vi "Begin.vi"(8 "error in":errorcluster) -> (0 "error out":errorcluster)   [LabVIEW 2014]
doc: "Called before other user functions, this VI is expected to open initial I/O refnums, load in file data, and do all program initialization. Notice that the <B>error out</B> terminal is simply used for data flow. Wiring it to other structures or subVIs ensures that this VI runs first."
uses:
  <vilib>/Rock Robotics/WPI/SafetyOutput/WPI_SafetyOutputConfigMenu.ctl
  <vilib>/Rock Robotics/WPI/DriverStation/WPI_DriverStationRobotMode2.ctl
  <vilib>/Rock Robotics/WPI/Joystick/WPI_JoystickDeviceEnum.ctl
  <vilib>/Rock Robotics/SystemInterfaces/DIO/FPGA_DIOChannel.ctl
  <vilib>/Rock Robotics/WPI/CAN/Jaguar/SubVIs/WPI_CANJaguar_ControlMode.ctl
  <vilib>/Rock Robotics/WPI/Solenoid/WPI_SolenoidChannel.ctl
  <vilib>/Rock Robotics/SystemInterfaces/Typedef/FPGA_TypedefDigitalModule.ctl
  <vilib>/Rock Robotics/SystemInterfaces/DIO/FPGA_DIOPWMChannel.ctl
  Robot Global Data.vi
  <vilib>/Rock Robotics/Network Tables/SD Write String Array.vi
  <vilib>/Rock Robotics/WPI/RobotDrive/WPI_RobotDriveOpen4MotorWithCANTalonSRX.vi
  <vilib>/Utility/config.llb/Read Key (String).vi
  <vilib>/Rock Robotics/WPI/Counter/WPI_CounterDigitalInputToDigitalSource.vi
  <vilib>/Rock Robotics/WPI/MotorControl/WPI_MotorControlOpenCANJaguar.vi
  <vilib>/Rock Robotics/WPI/Switch/WPI_SwitchOpenLimit.vi
  <vilib>/Rock Robotics/WPI/Compressor/WPI_CompressorGetSetRefNum.vi
  <vilib>/Rock Robotics/WPI/Solenoid/WPI_SolenoidOpenDouble.vi
  <vilib>/Rock Robotics/WPI/Ultrasonic/WPI_SonarMB1010DigitalOpen.vi
  <vilib>/Rock Robotics/WPI/Ultrasonic/WPI_SonarMB1010DigRefNum Registry Set.vi
  <vilib>/Rock Robotics/WPI/MotorControl/WPI_MotorControlOpen VictorSP.vi
  <vilib>/Utility/config.llb/NI_LVConfig.lvlib
panel:
  out "1699-preferences.ini":string[][](array[string])
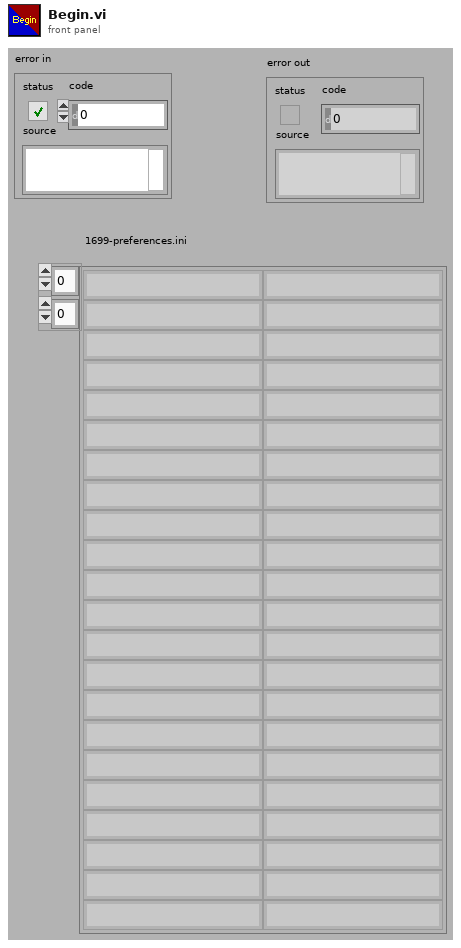
[diagram p1: front panel]
types:
  T1 = typedef "FPGA_DIOPWMChannel.ctl" = enum8{"PWM 0", "PWM 1", "PWM 2", "PWM 3", "PWM 4", "PWM 5", "PWM 6", "PWM 7", "PWM 8", "PWM 9", "PWM MXP 0", "PWM MXP 1", "PWM MXP 2", "PWM MXP 3", "PWM MXP 4", "PWM MXP 5", "PWM MXP 6", "PWM MXP 7", "PWM MXP 8", "PWM MXP 9", "Invalid"}
  T2 = typedef "FPGA_TypedefDigitalModule.ctl" = enum16{"Controller 1"}
  T3 = typedef "FPGA_DIOChannel.ctl" = enum8{"DIO 0", "DIO 1", "DIO 2", "DIO 3", "DIO 4", "DIO 5", "DIO 6", "DIO 7", "DIO 8", "DIO 9", "DIO MXP 0", "DIO MXP 1", "DIO MXP 2", "DIO MXP 3", "DIO MXP 4", "DIO MXP 5", "DIO MXP 6", "DIO MXP 7", "DIO MXP 8", "DIO MXP 9", "DIO MXP 10", "DIO MXP 11", "DIO MXP 12", "DIO MXP 13", "DIO MXP 14", "DIO MXP 15", "Invalid"}
  T4 = typedef "WPI_SolenoidChannel.ctl" = enum8{"Solenoid 0", "Solenoid 1", "Solenoid 2", "Solenoid 3", "Solenoid 4", "Solenoid 5", "Solenoid 6", "Solenoid 7", "Invalid"}
  T5 = typedef "WPI_CANJaguar_ControlMode.ctl" = enum8{"Percent VBus", "Current", "Speed", "Position", "Voltage"}
  T6 = typedef "WPI_JoystickDeviceEnum.ctl" = enum16{"USB 0", "USB 1", "USB 2", "USB 3", "USB 4", "USB 5"}
  T7 = typedef "WPI_DriverStationRobotMode2.ctl" = enum16{"Autonomous Disabled", "Autonomous Enabled", "Teleop Disabled", "Teleop Enabled", "Disconnected", "Finish", "Test Disabled", "Test Enabled", "Emergency Stopped"}
  T8 = typedef "WPI_SafetyOutputConfigMenu.ctl" = enum16{"Enable", "Disable"}
  T9 = typedef "NI_LVConfig.lvlib/Config Data RefNum.ctl" = refnum<k1>
  T10 = typedef "WPI_SolenoidDevRef.ctl" = cluster{"DevStatus":errorcluster, "Pneumatics Control Module":u8, "Forward Solenoid Channel":T4, "Reverse Solenoid Channel":T4}
  T11 = typedef "WPI_CompressorDevRef.ctl" = cluster{"DevStatus":errorcluster, "Pneumatics Control Module":u8}
  T12 = typedef "WPI_SwitchDevRef.ctl" = cluster{"DevStatus":errorcluster, "DIO Channel":T3, "Controller":T2, "CntIndex":T13, "Normally Closed":bool}
  T13 = typedef "FPGA_CounterCtrSystemIndex.ctl" = enum8{"Ctr 0", "Ctr 1", "Ctr 2", "Ctr 3", "Ctr 4", "Ctr 5", "Ctr 6", "Ctr 7", "Invalid"}
  T14 = typedef "WPI_SonarMB1010DigitalDeviceRef.ctl" = cluster{"CounterDevRef":T15, "Scaling factor (s/in)":dbl}
  T15 = typedef "WPI_CounterDevRef.ctl" = cluster{"DevStatus":errorcluster, "CntIndex":T13}
  T16 = typedef "WPI_MotorControlDeviceRef.ctl" = cluster{"DeviceStatus":errorcluster, "Type":T17, "PWM":cluster{"Controller":T2, "PWM Channel":T1, "DeadBand":T18}, "CAN":cluster{"Device Number":u8, "Control Mode":T5, "Semaphore":T19, "Max Vout":dbl, "TalonSRX Control Mode":T20}, "Invert":bool, "TransformRef":T21, "InvTransformRef":T21}
  T17 = typedef "WPI_MotorControlType.ctl" = enum16{"PWM", "CAN", "CANTalonSRX"}
  T18 = typedef "WPI_PWMDeadband.ctl" = cluster{"Name":string, "maxPositivePwm":i32, "minPositivePwm":i32, "centerPwm":i32, "maxNegativePwm":i32, "minNegativePwm":i32, "angularRange":u16}
  T19 = typedef "Semaphore RefNum" = refnum<k1>
  T20 = typedef "WPI_CANTalonSRX_APIControlMode.ctl" = enum8{"Percent VBus", "Speed", "Position", "Slave", "Unchanged / Invalid"}
  T21 = typedef "WPI_PWMTransform_ConPane.ctl" = refnum<vi>
  T22 = typedef "WPI_DigitalInputDevRef.ctl" = cluster{"DevStatus":errorcluster, "DIO Channel":T3, "Controller":T2}
  T23 = typedef "WPI_RobotDriveDevRef.ctl" = cluster{"DevStatus":errorcluster, "Motors[]":T16[], "Square Inputs":bool, "Max Output":dbl}
  T24 = typedef "WPI_JoystickDevRef.ctl" = cluster{"Device":T6}
  T25 = typedef "FPGA_CounterEncoderSourceConvertionLVSourceType.ctl" = cluster{"DevStatus":errorcluster, "AnalogTriggerMode?":bool, "DigitalMode":cluster{"Controller":T2, "DIO Channel":T26}, "AnalogTriggerMode":cluster{"AnalogTriggerIndex":T27, "OutputType":T28}}
  T26 = typedef "FPGA_DIODigitalSourceChannel.ctl" = enum8{"DIO 0", "DIO 1", "DIO 2", "DIO 3", "DIO 4", "DIO 5", "DIO 6", "DIO 7", "DIO 8", "DIO 9", "DIO MXP 0", "DIO MXP 1", "DIO MXP 2", "DIO MXP 3", "DIO MXP 4", "DIO MXP 5", "DIO MXP 6", "DIO MXP 7", "DIO MXP 8", "DIO MXP 9", "DIO MXP 10", "DIO MXP 11", "DIO MXP 12", "DIO MXP 13", "DIO MXP 14", "DIO MXP 15", "Disabled"}
  T27 = typedef "FPGA_AnalogTriggerIndex.ctl" = enum8{"Trig 0", "Trig 1", "Trig 2", "Trig 3", "Trig 4", "Trig 5", "Trig 6", "Trig 7", "Invalid"}
  T28 = typedef "FPGA_AnalogTriggerOutType.ctl" = enum16{"InWindow", "TriggerState", "Rising", "Falling"}
  T29 = cluster{"[0]":string, "[1]":string, "[2]":string, "[3]":string, "[4]":string, "[5]":string, "[6]":string, "[7]":string, "[8]":string, "[9]":string, "[10]":string, "[11]":string, "[12]":string, "[13]":string, "[14]":string, "[15]":string, "[16]":string, "[17]":string, "[18]":string, "[19]":string}
  T30 = typedef "WPI_EncoderDevRef.ctl" = cluster{"DevStatus":errorcluster, "EncoderIndex":T31, "CounterIndex":T13, "DistancePerCount":dbl, "Decoding Type":T32}
  T31 = typedef "FPGA_EncoderIdx.ctl" = enum8{"Enc 0", "Enc 1", "Enc 2", "Enc 3", "Enc 4", "Enc 5", "Enc 6", "Enc 7", "Invalid"}
  T32 = typedef "WPI_EncoderType.ctl" = enum16{"1x", "2x", "4x"}
  T33 = cluster{"[0]":dbl, "[1]":dbl, "[2]":dbl, "[3]":dbl, "[4]":dbl, "[5]":dbl, "[6]":dbl, "[7]":dbl, "[8]":dbl, "[9]":dbl, "[10]":dbl, "[11]":dbl, "[12]":dbl, "[13]":dbl, "[14]":dbl, "[15]":dbl, "[16]":dbl, "[17]":dbl, "[18]":dbl, "[19]":dbl}
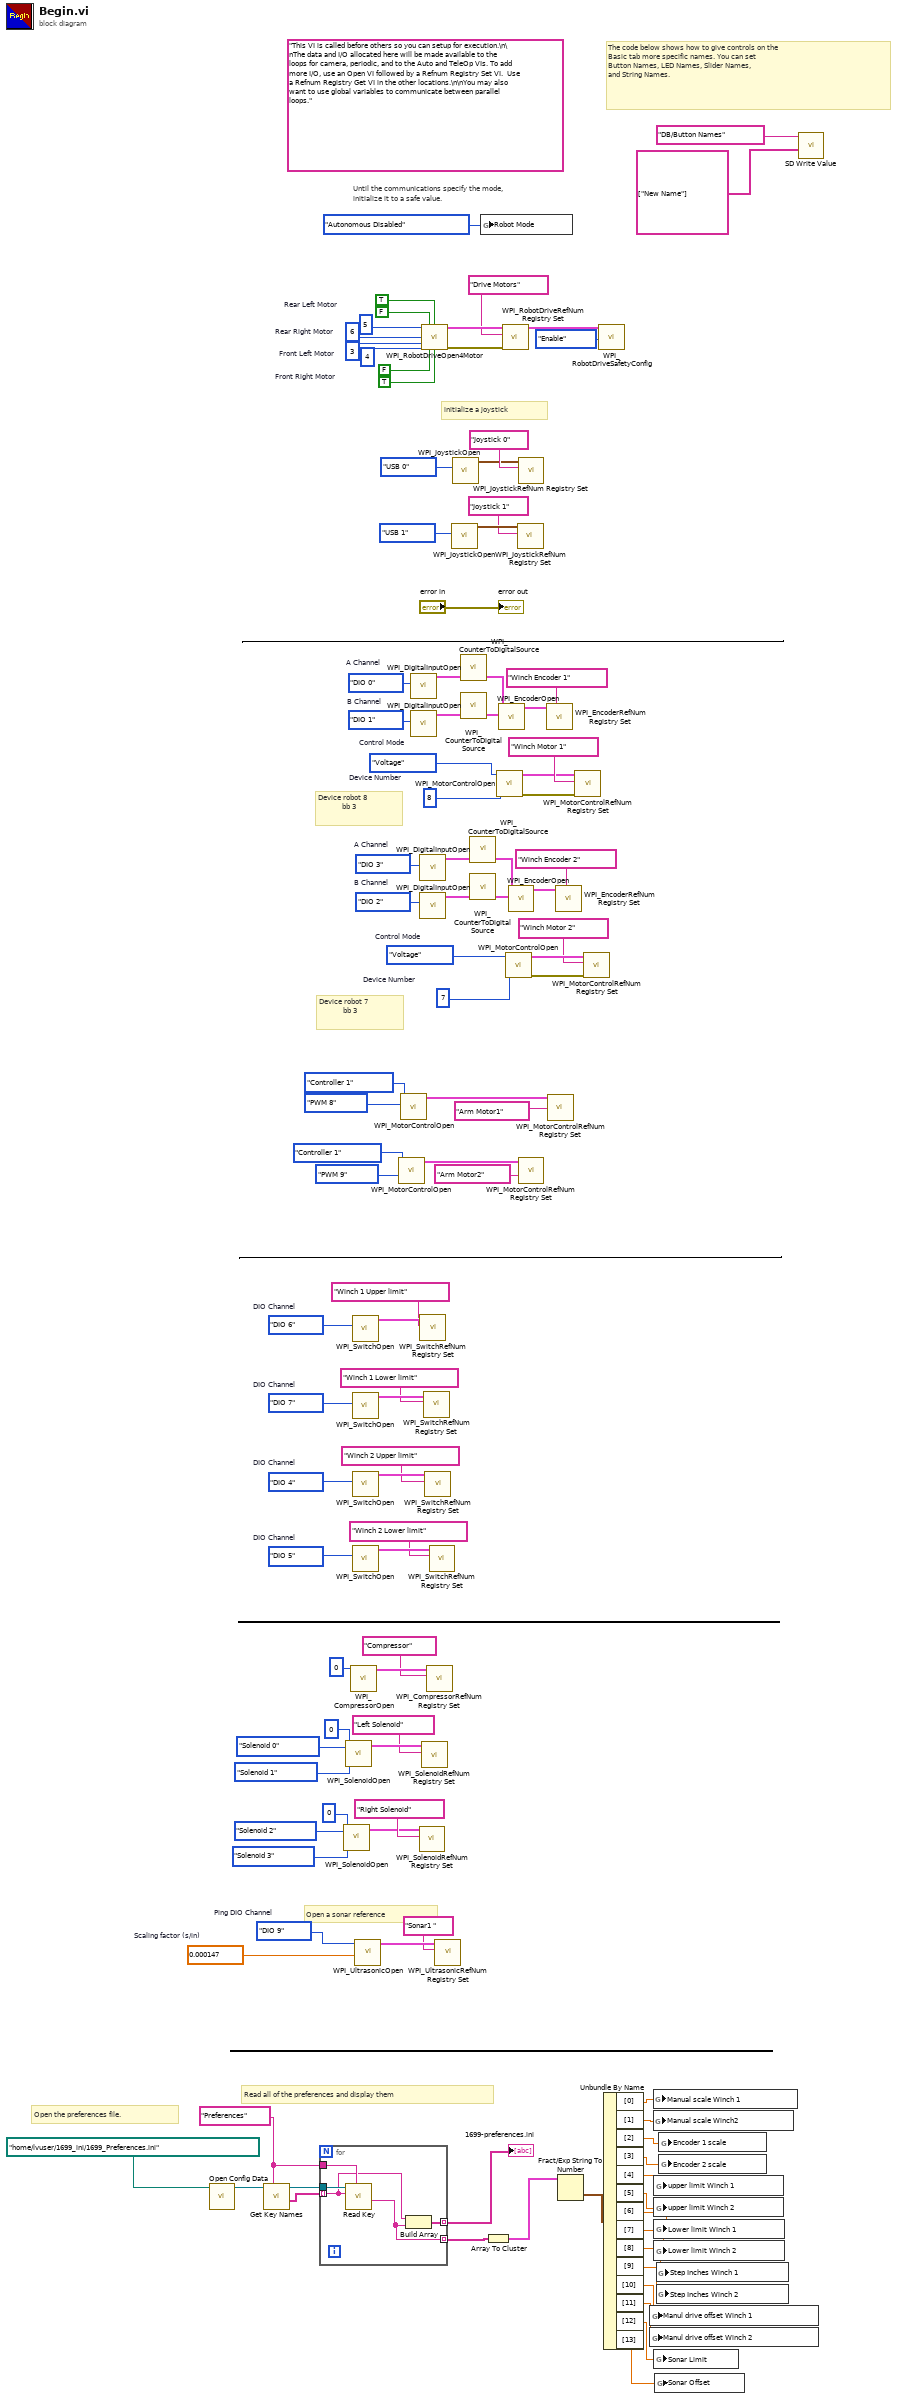
[diagram p0: block diagram]
diagram:
  w10 = 0.000147  # Scaling factor (s/in)
  w13 = FPGA_DIOChannel."DIO 9"  # Ping DIO Channel
  w30 = WPI_CANJaguar_ControlMode."Voltage"  # Control Mode
  w31 = u8 8  # Device Number
  w42 = FPGA_DIOChannel."DIO 1"  # B Channel
  w41 = FPGA_DIOChannel."DIO 0"  # A Channel
  w56 = FPGA_DIOChannel."DIO 5"  # DIO Channel
  w55 = FPGA_DIOChannel."DIO 4"  # DIO Channel
  w54 = FPGA_DIOChannel."DIO 7"  # DIO Channel
  w57 = FPGA_DIOChannel."DIO 6"  # DIO Channel
  w58 = u8 7  # Device Number
  w59 = WPI_CANJaguar_ControlMode."Voltage"  # Control Mode
  w60 = FPGA_DIOChannel."DIO 2"  # B Channel
  w61 = FPGA_DIOChannel."DIO 3"  # A Channel
  w77 = "Preferences" ("section")
  w92 = u8 4  # Front Right Motor
  w93 = u8 3  # Front Left Motor
  w94 = u8 6  # Rear Right Motor
  w95 = u8 5  # Rear Left Motor
  (unwired) "This VI is called before others so you can setup for execution.\n\nThe data and I/O allocated here will be made available to the loops for camera, periodic, and to the Auto and TeleOp VIs. To add more I/O, use an Open VI followed by a Refnum Registry Set VI.  Use a Refnum Registry Get VI in the other locations.\n\nYou may also want to use global variables to communicate between parallel loops."
  # "Device robot 7\n            bb 3"
  # "Device robot 8\n            bb 3"
  # "Open a sonar reference"
  # "Read all of the preferences and display them"
  # "Open the preferences file."
  # "The code below shows how to give controls on the\nBasic tab more specific names. You can set\nButton Names, LED Names, Slider Names,\nand String Names."
  # "initialize a joystick"
  # "Until the communications specify the mode,\ninitialize it to a safe value."
  n1 = call <vilib>:"Open Config Data.vi"("configuration file path"=path "/home/lvuser/1699_ini/1699_Preferences.ini") -> ("refnum"=w79:T9)  [unwired: 8 in, 2 out]
  n2 = call <vilib>:"Get Key Names.vi"("section"=w77, "refnum"=w79) -> ("key names"=w78:string[], "refnum out"=w76:T9)  [unwired: 6 in, 2 out]
  n3 = for {
    tunnel: w78 -> [w112] mode=indexing
    tunnel: w76 -> [w114]
    tunnel: w77 -> [w113]
    tunnel: [w111] -> w72 mode=indexing
    tunnel: [w110] -> w74 mode=indexing
    n4 = call-poly <vilib>:"Read Key.vi"("section"=w113, "key"=w112, "refnum"=w114) -> ("value"=w110:string)  [unwired: 5 in, 3 out]
    n5 = Build Array(w112, w110) -> (w111:string[])
  }
  "1699-preferences.ini" <- w72
  n6 = call-poly <vilib>:"WPI_SolenoidOpen.vi"("Reverse Solenoid Channel"=WPI_SolenoidChannel."Solenoid 3", "Forward Solenoid Channel"=WPI_SolenoidChannel."Solenoid 2", "Pneumatics Control Module (0)"=u8 0) -> ("SolenoidDevRef"=w20:T10)  [unwired: 7 in, 1 out]
  n7 = call-poly <vilib>:"WPI_SolenoidOpen.vi"("Reverse Solenoid Channel"=WPI_SolenoidChannel."Solenoid 1", "Forward Solenoid Channel"=WPI_SolenoidChannel."Solenoid 0", "Pneumatics Control Module (0)"=u8 0) -> ("SolenoidDevRef"=w23:T10)  [unwired: 7 in, 1 out]
  n8 = call <vilib>:"WPI_CompressorOpen.vi"("Pneumatics Control Module (0)"=u8 0) -> ("CompressorDevRef"=w28:T11)  [unwired: 13 in, 1 out]
  n9 = call-poly <vilib>:"WPI_SwitchOpen.vi"("DIO Channel"=w57) -> ("SwitchDevRef"=w50:T12)  [unwired: 9 in, 1 out]
  n10 = call-poly <vilib>:"WPI_SwitchOpen.vi"("DIO Channel"=w54) -> ("SwitchDevRef"=w51:T12)  [unwired: 9 in, 1 out]
  n11 = call-poly <vilib>:"WPI_SwitchOpen.vi"("DIO Channel"=w55) -> ("SwitchDevRef"=w52:T12)  [unwired: 9 in, 1 out]
  n12 = call-poly <vilib>:"WPI_SwitchOpen.vi"("DIO Channel"=w56) -> ("SwitchDevRef"=w53:T12)  [unwired: 9 in, 1 out]
  n13 = call-poly <vilib>:"WPI_UltrasonicOpen.vi"("Scaling factor (s/in)"=w10, "DIO Channel"=w13) -> ("SonarMB1010DigitalDevRef"=w12:T14)  [unwired: 8 in, 1 out]
  n14 = call-poly <vilib>:"WPI_MotorControlOpen.vi"("PWM Channel"=FPGA_DIOPWMChannel."PWM 9", "Controller"=FPGA_TypedefDigitalModule."Controller 1") -> ("MotorControlDeviceRef"=w7:T16)  [unwired: 8 in, 1 out]
  n15 = call-poly <vilib>:"WPI_MotorControlOpen.vi"("PWM Channel"=FPGA_DIOPWMChannel."PWM 8", "Controller"=FPGA_TypedefDigitalModule."Controller 1") -> ("MotorControlDeviceRef"=w8:T16)  [unwired: 8 in, 1 out]
  n16 = call <vilib>:"WPI_DigitalInputOpen.vi"("DIO Channel"=w41) -> ("DigitalInputDevRef"=w38:T22)  [unwired: 2 in, 8 out]
  n17 = call <vilib>:"WPI_DigitalInputOpen.vi"("DIO Channel"=w42) -> ("DigitalInputDevRef"=w39:T22)  [unwired: 2 in, 8 out]
  n18 = call <vilib>:"WPI_SolenoidRefNum Registry Set.vi"("refnum name"="Right Solenoid", "SolenoidDevRef"=w20) -> ()  [unwired: 8 in, 2 out]
  n19 = call <vilib>:"WPI_DigitalInputOpen.vi"("DIO Channel"=w61) -> ("DigitalInputDevRef"=w64:T22)  [unwired: 2 in, 8 out]
  n20 = call <vilib>:"WPI_DigitalInputOpen.vi"("DIO Channel"=w60) -> ("DigitalInputDevRef"=w63:T22)  [unwired: 2 in, 8 out]
  n21 = call <vilib>:"WPI_SwitchRefNum Registry Set.vi"("refnum name"="Winch 1 Upper limit", "SwitchDevRef"=w50) -> ()  [unwired: 8 in, 2 out]
  n22 = call-poly <vilib>:"WPI_RobotDriveOpen4Motor.vi"("Rear Left Motor"=w95, "Rear Left Motor Inverted"=FALSE, "Rear Right Motor Inverted"=TRUE, "Rear Right Motor"=w94, "Front Left Motor"=w93, "Front Right Motor"=w92, "Front Left Motor Inverted"=FALSE, "Front Right Motor Inverted"=TRUE) -> ("RobotDriveDevRef"=w107:T23, "error out"=w105:errorcluster)  [unwired: 6 in]
  n23 = call <vilib>:"WPI_SolenoidRefNum Registry Set.vi"("refnum name"="Left Solenoid", "SolenoidDevRef"=w23) -> ()  [unwired: 8 in, 2 out]
  n24 = call <vilib>:"WPI_SwitchRefNum Registry Set.vi"("refnum name"="Winch 1 Lower limit", "SwitchDevRef"=w51) -> ()  [unwired: 8 in, 2 out]
  n25 = call <vilib>:"WPI_SwitchRefNum Registry Set.vi"("refnum name"="Winch 2 Upper limit", "SwitchDevRef"=w52) -> ()  [unwired: 8 in, 2 out]
  n26 = call <vilib>:"WPI_CompressorRefNum Registry Set.vi"("refnum name"="Compressor", "CompressorDevRef"=w28) -> ()  [unwired: 8 in, 2 out]
  n27 = call <vilib>:"WPI_SwitchRefNum Registry Set.vi"("refnum name"="Winch 2 Lower limit", "SwitchDevRef"=w53) -> ()  [unwired: 8 in, 2 out]
  n28 = call-poly <vilib>:"WPI_UltrasonicRefNum Registry Set.vi"("refnum name"="Sonar1 ", "SonarMB1010DigitalDevRef"=w12) -> ()  [unwired: 8 in, 2 out]
  n29 = call <vilib>:"WPI_JoystickOpen.vi"("JoystickDevice"=WPI_JoystickDeviceEnum."USB 1") -> ("JoystickDevRef"=w44:T24)  [unwired: 10 in]
  n30 = call <vilib>:"WPI_JoystickOpen.vi"("JoystickDevice"=WPI_JoystickDeviceEnum."USB 0") -> ("JoystickDevRef"=w100:T24)  [unwired: 10 in]
  n31 = call-poly <vilib>:"WPI_CounterToDigitalSource.vi"("DigitalInputDevRef"=w38) -> ("Digital Source"=w37:T25)  [unwired: 6 out]
  n32 = call-poly <vilib>:"WPI_CounterToDigitalSource.vi"("DigitalInputDevRef"=w39) -> ("Digital Source"=w40:T25)  [unwired: 6 out]
  n33 = call-poly <vilib>:"WPI_CounterToDigitalSource.vi"("DigitalInputDevRef"=w64) -> ("Digital Source"=w65:T25)  [unwired: 6 out]
  n34 = call-poly <vilib>:"WPI_CounterToDigitalSource.vi"("DigitalInputDevRef"=w63) -> ("Digital Source"=w62:T25)  [unwired: 6 out]
  n35 = global write "Robot Global Data.vi" "Robot Mode"(WPI_DriverStationRobotMode2."Autonomous Disabled" ("Robot Mode")) -> ()
  n36 = Array To Cluster(array=w74) -> (cluster=w75:T29)
  n37 = call-poly <vilib>:"WPI_MotorControlOpen.vi"("Device Number"=w31, "Control Mode"=w30) -> ("error out"=w32:errorcluster, "MotorControlDeviceRef"=w33:T16)  [unwired: 8 in]
  n38 = call <vilib>:"WPI_EncoderOpen.vi"("BSource"=w40, "ASource"=w37) -> ("EncoderDevRef"=w36:T30)  [unwired: 6 in, 3 out]
  n39 = call <vilib>:"WPI_RobotDriveRefNum Registry Set.vi"("error in (no error)"=w105, "refnum name"="Drive Motors", "RobotDriveDevRef"=w107) -> ("RobotDriveDevRef"=w104:T23)  [unwired: 8 out]
  n40 = call-poly <vilib>:"WPI_MotorControlOpen.vi"("Device Number"=w58, "Control Mode"=w59) -> ("error out"=w70:errorcluster, "MotorControlDeviceRef"=w69:T16)  [unwired: 8 in]
  n41 = call <vilib>:"WPI_EncoderOpen.vi"("BSource"=w62, "ASource"=w65) -> ("EncoderDevRef"=w66:T30)  [unwired: 6 in, 3 out]
  n42 = call <vilib>:"WPI_JoystickRefNum Registry Set.vi"("refnum name"="Joystick 1", "JoystickDevRef"=w44) -> ()  [unwired: 8 in, 2 out]
  n43 = call <vilib>:"WPI_JoystickRefNum Registry Set.vi"("refnum name"="Joystick 0", "JoystickDevRef"=w100) -> ()  [unwired: 8 in, 2 out]
  n44 = call <vilib>:"WPI_MotorControlRefNum Registry Set.vi"("refnum name"="Arm Motor2", "MotorControlDevRef"=w7) -> ()  [unwired: 8 in, 2 out]
  n45 = call <vilib>:"WPI_EncoderRefNum Registry Set.vi"("refnum name"="Winch Encoder 1", "EncoderDevRef"=w36) -> ()  [unwired: 8 in, 2 out]
  n46 = call <vilib>:"WPI_MotorControlRefNum Registry Set.vi"("refnum name"="Arm Motor1", "MotorControlDevRef"=w8) -> ()  [unwired: 8 in, 2 out]
  n47 = call <vilib>:"WPI_EncoderRefNum Registry Set.vi"("refnum name"="Winch Encoder 2", "EncoderDevRef"=w66) -> ()  [unwired: 8 in, 2 out]
  n48 = Fract/Exp String To Number(string=w75) -> (number=w73:T33)  [unwired: 3 in, 1 out]
  n49 = call <vilib>:"WPI_MotorControlRefNum Registry Set.vi"("error in (no error)"=w32, "refnum name"="Winch Motor 1", "MotorControlDevRef"=w33) -> ()  [unwired: 7 in, 2 out]
  n50 = call <vilib>:"WPI_MotorControlRefNum Registry Set.vi"("error in (no error)"=w70, "refnum name"="Winch Motor 2", "MotorControlDevRef"=w69) -> ()  [unwired: 7 in, 2 out]
  n51 = call <vilib>:"WPI_RobotDriveSafetyConfig.vi"("mode"=WPI_SafetyOutputConfigMenu."Enable", "RobotDriveDevRef"=w104) -> ()  [unwired: 8 in, 2 out]
  n52 = Unbundle By Name(w73) -> ("[0]"=w89:dbl, "[1]"=w88:dbl, "[2]"=w87:dbl, "[3]"=w86:dbl, "[4]"=w85:dbl, "[5]"=w84:dbl, "[6]"=w83:dbl, "[7]"=w82:dbl, "[8]"=w81:dbl, "[9]"=w80:dbl, "[10]"=w16:dbl, "[11]"=w15:dbl, "[12]"=w14:dbl, "[13]"=w9:dbl)
  n53 = global write "Robot Global Data.vi" "Manul drive offset Winch 1"(w16) -> ()
  n54 = global write "Robot Global Data.vi" "Manul drive offset Winch 2"(w15) -> ()
  n55 = global write "Robot Global Data.vi" "Manual scale Winch 1"(w89) -> ()
  n56 = global write "Robot Global Data.vi" "Manual scale Winch2"(w88) -> ()
  n57 = global write "Robot Global Data.vi" "upper limit Winch 1"(w85) -> ()
  n58 = global write "Robot Global Data.vi" "upper limit Winch 2"(w84) -> ()
  n59 = global write "Robot Global Data.vi" "Lower limit Winch 1"(w83) -> ()
  n60 = global write "Robot Global Data.vi" "Lower limit Winch 2"(w82) -> ()
  n61 = global write "Robot Global Data.vi" "Sonar Limit"(w14) -> ()
  n62 = global write "Robot Global Data.vi" "Sonar Offset"(w9) -> ()
  n63 = global write "Robot Global Data.vi" "Step Inches Winch 1"(w81) -> ()
  n64 = global write "Robot Global Data.vi" "Step Inches Winch 2"(w80) -> ()
  n65 = global write "Robot Global Data.vi" "Encoder 1 scale"(w87) -> ()
  n66 = global write "Robot Global Data.vi" "Encoder 2 scale"(w86) -> ()
  n67 = call-poly <vilib>:"SD Write Value.vi"("String Array"=string[] ["New Name"], "Name"="DB/Button Names") -> ()  [unwired: 8 in, 2 out]
  "error out" <- "error in"
